vi "SW_Debounce_filter_U16.vi"() -> ()   [LabVIEW 2016]
panel:
  out "\"Debounced\" output":u16
  in  "Input":u16
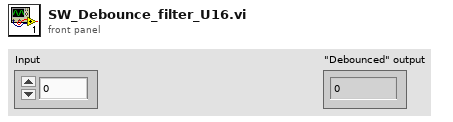
[diagram p1: front panel]
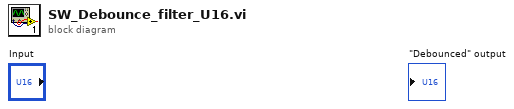
[diagram p0: block diagram]
diagram:
